vi "Configure RAMP DOWN.vi"(7 "All Channels (F)":bool, 8 "error in (no error)":errorcluster, 9 "Voltage ramp down (0 V/s)":u16 max=999, 10 "Channel (0)":u8, 11 "BoardHandle":T1) -> (0 "error out":errorcluster, 3 "BoardHandle out":T1)   [LabVIEW 2020, in "CAEN PSM.lvlib"]
doc: "This function allows to configure Voltage Ramp Down rate."
uses:
  CAEN PSM.lvlib
  Private/BoardHandle.ctl
  Private/DeviceFamily.ctl
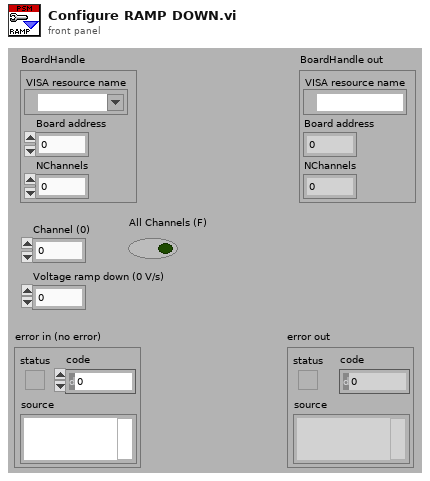
[diagram p1: front panel]
types:
  T1 = typedef "CAEN PSM.lvlib/BoardHandle.ctl" = cluster{"VISA resource name":refnum<visa-resource-name>, "Board address":i8, "NChannels":u8}
  T2 = typedef "CAEN PSM.lvlib/DeviceFamily.ctl" = enum8{"NIM / DESKTOP HV", "DT55XXE HV", "SMART HV"}
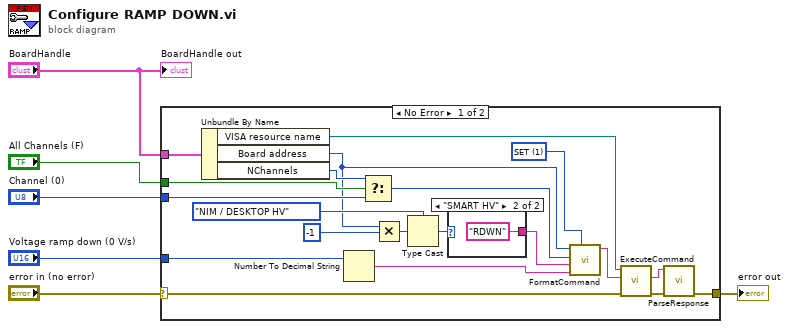
[diagram p0: block diagram]
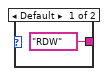
[diagram p2: hidden frame]
diagram:
  n1 = case shown="No Error" "error in (no error)" {
    selector: "error in (no error)" -> [w15 w29]
    tunnel: "All Channels (F)" -> [w25 _]
    tunnel: "Channel (0)" -> [w23 _]
    tunnel: [w18 w29] -> w3
    tunnel: "BoardHandle" -> [w16 _]
    tunnel: "Voltage ramp down (0 V/s)" -> [w14 _]
    frame No Error {
      w26 = u8 1 items=["MON", "SET"] ("CMD")
      n2 = Unbundle By Name(w16) -> ("VISA resource name"=w21:refnum<visa-resource-name>, "Board address"=w9:i8, "NChannels"=w24:u8)
      n3 = Number To Decimal String(number=w14) -> (decimal integer string=w13:string)  [unwired: 1 in]
      n4 = Select(t=w24, s=w25, f=w23) -> (s? t:f=w22:u8)
      n5 = Multiply(x=w9, y=i8 -1 ("x")) -> (x*y=w10:i8)
      n6 = Type Cast(type=DeviceFamily."NIM / DESKTOP HV" ("Device Family"), x=w10) -> (*(type *) &x=w12:T2)
      n7 = case shown="\"SMART HV\"" w12 {
        tunnel: ["RDW" ("PAR") "RDWN" ("PAR")] -> w7
        frame Default {
        }
        frame "SMART HV" {
        }
      }
      n8 = call "FormatCommand.vi"("CMD (MON)"=w26, "VAL"=w13, "PAR"=w7, "CH"=w22, "BD (0)"=w9) -> ("cmd"=w20:string)  [unwired: 6 in]
      n9 = call "ExecuteCommand.vi"("error in (no error)"=w15, "Command"=w20, "VISA resource name"=w21) -> ("error out"=w19:errorcluster, "Response"=w17:string)  [unwired: 6 in, 1 out]
      n10 = call "ParseResponse.vi"("error in (no error)"=w19, "Response"=w17) -> ("error out"=w18:errorcluster)  [unwired: 6 in, 3 out]
    }
    frame Error {
    }
  }
  "error out" <- w3
  "BoardHandle out" <- "BoardHandle"
